vi "data_waypoint_ref.vi"() -> ()   [LabVIEW 2018] (continued)
"Y"=530253.3628541183}, {"X"=175364.75731318252, "Y"=530253.4135907482}, {"X"=175364.79603092565, "Y"=530253.4635879273}, {"X"=175364.8341888009, "Y"=530253.5129652326}, {"X"=175364.8714835971, "Y"=530253.5616292221}, {"X"=175364.90849024183, "Y"=530253.6105027163}, {"X"=175364.94563348373, "Y"=530253.6594390685}, {"X"=175364.98314331504, "Y"=530253.7089359304}, {"X"=175365.02100005752, "Y"=530253.7595272006}, {"X"=175365.05918145005, "Y"=530253.8114759818}, {"X"=175365.09803261896, "Y"=530253.864670273}, {"X"=175365.1369677881, "Y"=530253.9178143732}, {"X"=175365.175450904, "Y"=530253.9711551395}, {"X"=175365.2146263419, "Y"=530254.0234727964}, {"X"=175365.25404981908, "Y"=530254.0748962869}, {"X"=175365.29313406267, "Y"=530254.1257247813}, {"X"=175365.3311370293, "Y"=530254.1760414864}, {"X"=175365.36840857498, "Y"=530254.2258364942}, {"X"=175365.40494955413, "Y"=530254.2744971587}, {"X"=175365.44107322232, "Y"=530254.3225197739}, {"X"=175365.4766030218, "Y"=530254.3695064213}, {"X"=175365.51182505823, "Y"=530254.4166593428}, {"X"=175365.54752247653, "Y"=530254.4640172995}, {"X"=175365.58419388309, "Y"=530254.5115499632}, {"X"=175365.62093701866, "Y"=530254.5602788435}, {"X"=175365.65774631436, "Y"=530254.6098177265}, {"X"=175365.6950449408, "Y"=530254.6597857933}, {"X"=175365.73257001908, "Y"=530254.7099496393}, {"X"=175365.76995592058, "Y"=530254.7600772697}, {"X"=175365.80677752316, "Y"=530254.8101854757}, {"X"=175365.84416599848, "Y"=530254.8596838082}, {"X"=175365.88176222175, "Y"=530254.9096443404}, {"X"=175365.91953173553, "Y"=530254.9594944854}, {"X"=175365.9574402241, "Y"=530255.0090134849}, {"X"=175365.99470143978, "Y"=530255.0589117429}, {"X"=175366.03154062154, "Y"=530255.1089755029}, {"X"=175366.0680535847, "Y"=530255.1592533174}, {"X"=175366.10490100825, "Y"=530255.2091083997}, {"X"=175366.1418778741, "Y"=530255.2596034913}, {"X"=175366.1794578632, "Y"=530255.3106683819}, {"X"=175366.2173681856, "Y"=530255.3620142048}, {"X"=175366.25529422174, "Y"=530255.4138827252}, {"X"=175366.29256422166, "Y"=530255.465561172}, {"X"=175366.3293060358, "Y"=530255.517452049}, {"X"=175366.36565792985, "Y"=530255.5689833704}, {"X"=175366.40203412157, "Y"=530255.6200418209}, {"X"=175366.4388502521, "Y"=530255.6703997643}, {"X"=175366.47596965497, "Y"=530255.7205714668}, {"X"=175366.51282475406, "Y"=530255.770928185}, {"X"=175366.5496163633, "Y"=530255.821080876}, {"X"=175366.58622919343, "Y"=530255.8712851491}, {"X"=175366.62272470424, "Y"=530255.9216551357}, {"X"=175366.65895272506, "Y"=530255.9726318942}, {"X"=175366.69602994501, "Y"=530256.0244207871}, {"X"=175366.73390271078, "Y"=530256.0771507177}, {"X"=175366.77233000507, "Y"=530256.1316958538}, {"X"=175366.81173351035, "Y"=530256.1868696233}, {"X"=175366.8519770966, "Y"=530256.2427678755}, {"X"=175366.8918884384, "Y"=530256.2989401333}, {"X"=175366.93135789846, "Y"=530256.3554544192}, {"X"=175366.9706897959, "Y"=530256.4115784413}, {"X"=175367.01058779864, "Y"=530256.4677340913}, {"X"=175367.05065983246, "Y"=530256.5246328339}, {"X"=175367.09101690596, "Y"=530256.5811689214}, {"X"=175367.1310731591, "Y"=530256.6375227704}, {"X"=175367.17083612958, "Y"=530256.6932448632}, {"X"=175367.21025581684, "Y"=530256.7481999461}, {"X"=175367.2492354851, "Y"=530256.8023261506}, {"X"=175367.287581066, "Y"=530256.8564975066}, {"X"=175367.32615449073, "Y"=530256.910735893}, {"X"=175367.3651370734, "Y"=530256.9652505389}, {"X"=175367.40405244404, "Y"=530257.0192004658}, {"X"=175367.44224889282, "Y"=530257.0729627243}, {"X"=175367.48063509667, "Y"=530257.1270928971}, {"X"=175367.5193307458, "Y"=530257.1810268238}, {"X"=175367.55835376275, "Y"=530257.2354370258}, {"X"=175367.59777806984, "Y"=530257.2904586872}, {"X"=175367.63832748993, "Y"=530257.3464415018}, {"X"=175367.67939942481, "Y"=530257.4029932447}, {"X"=175367.7207491782, "Y"=530257.4600391674}, {"X"=175367.7617005033, "Y"=530257.5171439771}, {"X"=175367.80307118673, "Y"=530257.5743796235}, {"X"=175367.84486851882, "Y"=530257.6312133558}, {"X"=175367.88690845872, "Y"=530257.6877145241}, {"X"=175367.92825091735, "Y"=530257.7446905482}, {"X"=175367.9699223432, "Y"=530257.8011817061}, {"X"=175368.01151293772, "Y"=530257.8572957474}, {"X"=175368.05314487906, "Y"=530257.9130123383}, {"X"=175368.09419173302, "Y"=530257.9685697247}, {"X"=175368.13502857919, "Y"=530258.0240999819}, {"X"=175368.17578947498, "Y"=530258.0794073816}, {"X"=175368.21706993572, "Y"=530258.1336810826}, {"X"=175368.2580036735, "Y"=530258.1878248417}, {"X"=175368.29871781138, "Y"=530258.2416928933}, {"X"=175368.33960146687, "Y"=530258.29567476}, {"X"=175368.38056272513, "Y"=530258.349538754}, {"X"=175368.42160467047, "Y"=530258.403431366}, {"X"=175368.46324653408, "Y"=530258.4574065608}, {"X"=175368.50493600065, "Y"=530258.5113039257}, {"X"=175368.546039586, "Y"=530258.5653739354}, {"X"=175368.58627301786, "Y"=530258.619636295}, {"X"=175368.62661766922, "Y"=530258.6737673621}, {"X"=175368.66737663423, "Y"=530258.7275187485}, {"X"=175368.707789486, "Y"=530258.7819492777}, {"X"=175368.74817281184, "Y"=530258.8368815499}, {"X"=175368.78905969212, "Y"=530258.8922607239}, {"X"=175368.83060171016, "Y"=530258.9472239888}, {"X"=175368.87236381875, "Y"=530259.0017271258}, {"X"=175368.91362172773, "Y"=530259.0555647215}, {"X"=175368.9541187612, "Y"=530259.1088041244}, {"X"=175368.99351905257, "Y"=530259.161693824}, {"X"=175369.03251394143, "Y"=530259.2140797316}, {"X"=175369.07165795774, "Y"=530259.2668725194}, {"X"=175369.1116919916, "Y"=530259.3202020752}, {"X"=175369.1522712206, "Y"=530259.3739828493}, {"X"=175369.19244677763, "Y"=530259.4275450595}, {"X"=175369.2315454748, "Y"=530259.4811925745}, {"X"=175369.27035327113, "Y"=530259.5341139864}, {"X"=175369.30912567972, "Y"=530259.5858479531}, {"X"=175369.34761534786, "Y"=530259.637222049}, {"X"=175369.38570391198, "Y"=530259.6883464997}, {"X"=175369.4236531108, "Y"=530259.7393714729}, {"X"=175369.4617789277, "Y"=530259.7896123657}, {"X"=175369.49993611278, "Y"=530259.8390751553}, {"X"=175369.53771359075, "Y"=530259.8880362958}, {"X"=175369.57511864332, "Y"=530259.9371627924}, {"X"=175369.61242632216, "Y"=530259.9872129811}, {"X"=175369.65026476423, "Y"=530260.0379253004}, {"X"=175369.68844804208, "Y"=530260.0899329198}, {"X"=175369.72774864096, "Y"=530260.1420593341}, {"X"=175369.76747697193, "Y"=530260.1944530737}, {"X"=175369.80690045215, "Y"=530260.2470996501}, {"X"=175369.84600582987, "Y"=530260.2994086567}, {"X"=175369.8855787249, "Y"=530260.3516585723}, {"X"=175369.92548969664, "Y"=530260.4038098247}, {"X"=175369.96521553188, "Y"=530260.4568606102}, {"X"=175370.0048233524, "Y"=530260.5098418208}, {"X"=175370.04435833584, "Y"=530260.5630540976}, {"X"=175370.08360233658, "Y"=530260.6155147478}, {"X"=175370.12268043496, "Y"=530260.6666828998}, {"X"=175370.161077391, "Y"=530260.7169574014}, {"X"=175370.1988345409, "Y"=530260.7665367983}, {"X"=175370.23621340372, "Y"=530260.8160973303}, {"X"=175370.2741603868, "Y"=530260.8651700723}, {"X"=175370.31198308783, "Y"=530260.9147526048}, {"X"=175370.3494809023, "Y"=530260.9653027819}, {"X"=175370.38678381703, "Y"=530261.0161443175}, {"X"=175370.42433720775, "Y"=530261.0678208391}, {"X"=175370.4626341092, "Y"=530261.1193120438}, {"X"=175370.50168795633, "Y"=530261.1715712609}, {"X"=175370.54076009642, "Y"=530261.2252288469}, {"X"=175370.58048902013, "Y"=530261.279631433}, {"X"=175370.62107124308, "Y"=530261.333832843}, {"X"=175370.66210860672, "Y"=530261.3879840766}, {"X"=175370.70264565348, "Y"=530261.4421856187}, {"X"=175370.74249817466, "Y"=530261.4961483381}, {"X"=175370.78169428193, "Y"=530261.5497933521}, {"X"=175370.82119589235, "Y"=530261.6028059552}, {"X"=175370.8604972166, "Y"=530261.6560855159}, {"X"=175370.89999125095, "Y"=530261.7092335463}, {"X"=175370.93876096676, "Y"=530261.7621650669}, {"X"=175370.97771263926, "Y"=530261.8146221417}, {"X"=175371.01739352918, "Y"=530261.8662513338}, {"X"=175371.057154059, "Y"=530261.9175528833}, {"X"=175371.09605709632, "Y"=530261.9691366423}, {"X"=175371.13461257404, "Y"=530262.0218090902}, {"X"=175371.17493162048, "Y"=530262.074476341}, {"X"=175371.2161687712, "Y"=530262.1281930344}, {"X"=175371.2574986481, "Y"=530262.1824155508}, {"X"=175371.29896848748, "Y"=530262.2372436394}, {"X"=175371.34017383057, "Y"=530262.2927928045}, {"X"=175371.38163837852, "Y"=530262.3479305593}, {"X"=175371.4233859332, "Y"=530262.4026168778}, {"X"=175371.4653806578, "Y"=530262.457616558}, {"X"=175371.50709616198, "Y"=530262.5134505647}, {"X"=175371.5492311775, "Y"=530262.5688660291}, {"X"=175371.59135206408, "Y"=530262.6242970738}, {"X"=175371.63361993022, "Y"=530262.6797065984}, {"X"=175371.67533013487, "Y"=530262.7352465111}, {"X"=175371.7166030467, "Y"=530262.7908820468}, {"X"=175371.7576439664, "Y"=530262.846846788}, {"X"=175371.79961031346, "Y"=530262.9018365643}, {"X"=175371.8417403082, "Y"=530262.9558502925}, {"X"=175371.88340146284, "Y"=530263.0091728515}, {"X"=175371.92439824372, "Y"=530263.0615795128}, {"X"=175371.96503316762, "Y"=530263.1135310883}, {"X"=175372.0052249805, "Y"=530263.1648058448}, {"X"=175372.04496494954, "Y"=530263.216047527}, {"X"=175372.08486382675, "Y"=530263.267409716}, {"X"=175372.12527531054, "Y"=530263.3195872516}, {"X"=175372.16591554228, "Y"=530263.3718373646}, {"X"=175372.20672269005, "Y"=530263.4245209418}, {"X"=175372.24767576595, "Y"=530263.4771275077}, {"X"=175372.28965336786, "Y"=530263.5290240761}, {"X"=175372.33110264182, "Y"=530263.5816868937}, {"X"=175372.3726853523, "Y"=530263.6348432075}, {"X"=175372.4151099726, "Y"=530263.6881424303}, {"X"=175372.45798269208, "Y"=530263.7411051576}, {"X"=175372.50007205043, "Y"=530263.7942555395}, {"X"=175372.5416247459, "Y"=530263.8474474571}, {"X"=175372.5829580622, "Y"=530263.9010406794}, {"X"=175372.62484024334, "Y"=530263.9542238587}, {"X"=175372.66669413337, "Y"=530264.0071252142}, {"X"=175372.70904192966, "Y"=530264.0599052535}, {"X"=175372.75097860975, "Y"=530264.112345775}, {"X"=175372.7924628684, "Y"=530264.1645578903}, {"X"=175372.8333104372, "Y"=530264.2162313784}, {"X"=175372.8738449646, "Y"=530264.2680833666}, {"X"=175372.91441410081, "Y"=530264.319957451}, {"X"=175372.9557862025, "Y"=530264.3719834397}, {"X"=175372.99767016945, "Y"=530264.4239701862}, {"X"=175373.03924414562, "Y"=530264.4765704875}, {"X"=175373.0804756962, "Y"=530264.529296102}, {"X"=175373.12245933426, "Y"=530264.5811404951}, {"X"=175373.1641074646, "Y"=530264.6327539145}, {"X"=175373.2048067197, "Y"=530264.6842968779}, {"X"=175373.245243158, "Y"=530264.7356275225}, {"X"=175373.28613031158, "Y"=530264.7872098872}, {"X"=175373.3268719919, "Y"=530264.8396239675}, {"X"=175373.36816244232, "Y"=530264.8921995794}, {"X"=175373.40948345076, "Y"=530264.9443233894}, {"X"=175373.45060314657, "Y"=530264.9963656624}, {"X"=175373.49133239881, "Y"=530265.0475689222}, {"X"=175373.53206551704, "Y"=530265.0985812743}, {"X"=175373.5723972954, "Y"=530265.1501674973}, {"X"=175373.6127379377, "Y"=530265.2029590018}, {"X"=175373.65307959612, "Y"=530265.2560956681}, {"X"=175373.6935509451, "Y"=530265.3090554855}, {"X"=175373.73412274377, "Y"=530265.3609340055}, {"X"=175373.7750503279, "Y"=530265.4118103823}, {"X"=175373.8156763603, "Y"=530265.4625544671}, {"X"=175373.85636513907, "Y"=530265.512649098}, {"X"=175373.8966237603, "Y"=530265.5631567544}, {"X"=175373.9368359794, "Y"=530265.6141495564}, {"X"=175373.97664394762, "Y"=530265.6659315486}, {"X"=175374.01652882574, "Y"=530265.7176611514}, {"X"=175374.0558253849, "Y"=530265.7696377665}, {"X"=175374.09546728528, "Y"=530265.8215756294}, {"X"=175374.1352996199, "Y"=530265.8735107117}, {"X"=175374.1753605969, "Y"=530265.9263862808}, {"X"=175374.21554098636, "Y"=530265.9792048966}, {"X"=175374.25634345112, "Y"=530266.0321115775}, {"X"=175374.29684755186, "Y"=530266.0847660915}, {"X"=175374.3370072678, "Y"=530266.1368822271}, {"X"=175374.37684985562, "Y"=530266.1883899836}, {"X"=175374.41664284474, "Y"=530266.2401997693}, {"X"=175374.45623583646, "Y"=530266.2926760602}, {"X"=175374.4957903801, "Y"=530266.3453322599}, {"X"=175374.53494277128, "Y"=530266.3985856391}, {"X"=175374.5738609444, "Y"=530266.4514124128}, {"X"=175374.61273645412, "Y"=530266.5035878264}, {"X"=175374.6511642197, "Y"=530266.5553183937}, {"X"=175374.68891586334, "Y"=530266.6066558418}, {"X"=175374.72739777548, "Y"=530266.6569223469}, {"X"=175374.7656299184, "Y"=530266.7065947026}, {"X"=175374.80313963493, "Y"=530266.7566920433}, {"X"=175374.8399778119, "Y"=530266.8064484142}, {"X"=175374.8766657008, "Y"=530266.8563062254}, {"X"=175374.91344849125, "Y"=530266.9059040511}, {"X"=175374.95023190015, "Y"=530266.9560135192}, {"X"=175374.98740198716, "Y"=530267.0068876502}, {"X"=175375.02601149524, "Y"=530267.0580716352}, {"X"=175375.06553802377, "Y"=530267.1114426706}, {"X"=175375.10591067414, "Y"=530267.1669876481}, {"X"=175375.146517546, "Y"=530267.2238637658}, {"X"=175375.1877406851, "Y"=530267.2809611515}, {"X"=175375.22830013547, "Y"=530267.3382780246}, {"X"=175375.26785239112, "Y"=530267.3949719046}, {"X"=175375.30721058228, "Y"=530267.4504355218}, {"X"=175375.34715167427, "Y"=530267.5053180757}, {"X"=175375.38706773933, "Y"=530267.5595225785}, {"X"=175375.4267418654, "Y"=530267.613685621}, {"X"=175375.46535510637, "Y"=530267.6676442431}, {"X"=175375.50396058234, "Y"=530267.7216716999}, {"X"=175375.54284507962, "Y"=530267.7750990131}, {"X"=175375.58147326022, "Y"=530267.8287157561}, {"X"=175375.61925587003, "Y"=530267.8830519565}, {"X"=175375.6576886122, "Y"=530267.9376803568}, {"X"=175375.69664500767, "Y"=530267.9926623688}, {"X"=175375.73603756493, "Y"=530268.0480681743}, {"X"=175375.77532893803, "Y"=530268.1040047903}, {"X"=175375.81435740308, "Y"=530268.1602995562}, {"X"=175375.85262212646, "Y"=530268.2171293042}, {"X"=175375.89158039243, "Y"=530268.2739503484}, {"X"=175375.93173150255, "Y"=530268.330970986}, {"X"=175375.97191079802, "Y"=530268.3882379278}, {"X"=175376.01228297348, "Y"=530268.4463333681}, {"X"=175376.05265943654, "Y"=530268.5043810724}, {"X"=175376.09293965067, "Y"=530268.562530056}, {"X"=175376.13402299516, "Y"=530268.6205878863}, {"X"=175376.17550761972, "Y"=530268.6789541855}, {"X"=175376.2171191087, "Y"=530268.7382901298}, {"X"=175376.25857909265, "Y"=530268.798215855}, {"X"=175376.30063365336, "Y"=530268.8576137554}, {"X"=175376.34250984906, "Y"=530268.9169023044}, {"X"=175376.38375533113, "Y"=530268.9761782852}, {"X"=175376.4239993277, "Y"=530269.0352652095}, {"X"=175376.46462206956, "Y"=530269.0942278227}, {"X"=175376.5061171255, "Y"=530269.1522278391}, {"X"=175376.5475091983, "Y"=530269.20984859}, {"X"=175376.58769639168, "Y"=530269.2676948581}, {"X"=175376.62757688668, "Y"=530269.3254665607}, {"X"=175376.667320457, "Y"=530269.3824628744}, {"X"=175376.70731428557, "Y"=530269.4393174993}, {"X"=175376.74719239495, "Y"=530269.495980459}, {"X"=175376.7866007532, "Y"=530269.5537480027}, {"X"=175376.82704140185, "Y"=530269.6116368113}, {"X"=175376.86867427992, "Y"=530269.6692157873}, {"X"=175376.91032201465, "Y"=530269.7264251373}, {"X"=175376.9512818232, "Y"=530269.7837452792}, {"X"=175376.99105095697, "Y"=530269.8410012267}, {"X"=175377.02996204546, "Y"=530269.8986514817}, {"X"=175377.06897030905, "Y"=530269.9562137703}, {"X"=175377.1089557823, "Y"=530270.0135423321}, {"X"=175377.14928842592, "Y"=530270.0708510028}, {"X"=175377.18985192844, "Y"=530270.1274475757}, {"X"=175377.2301206264, "Y"=530270.1834967455}, {"X"=175377.2706423454, "Y"=530270.2388393001}, {"X"=175377.31043959537, "Y"=530270.2942139549}, {"X"=175377.34961013673, "Y"=530270.3497336272}, {"X"=175377.38805029093, "Y"=530270.4062842885}, {"X"=175377.42698760645, "Y"=530270.4629167287}, {"X"=175377.4664671266, "Y"=530270.5195853052}, {"X"=175377.50645504915, "Y"=530270.5753411908}, {"X"=175377.5459466516, "Y"=530270.6313005314}, {"X"=175377.58575752817, "Y"=530270.6876951077}, {"X"=175377.62575899236, "Y"=530270.7447406121}, {"X"=175377.66585884744, "Y"=530270.8024117845}, {"X"=175377.70568216513, "Y"=530270.8603246126}, {"X"=175377.74558738028, "Y"=530270.9180740495}, {"X"=175377.7855966506, "Y"=530270.974763265}, {"X"=175377.82569728378, "Y"=530271.0302924092}, {"X"=175377.86556871625, "Y"=530271.084692392}, {"X"=175377.90532123862, "Y"=530271.1393202449}, {"X"=175377.94501325546, "Y"=530271.1944565923}, {"X"=175377.98486513883, "Y"=530271.2503405145}, {"X"=175378.02435570536, "Y"=530271.3062510273}, {"X"=175378.06409336728, "Y"=530271.3621497148}, {"X"=175378.103309077, "Y"=530271.4176703686}, {"X"=175378.14220560313, "Y"=530271.473087634}, {"X"=175378.1814429543, "Y"=530271.5284373041}, {"X"=175378.22134028416, "Y"=530271.5838127786}, {"X"=175378.26121354155, "Y"=530271.6397365938}, {"X"=175378.30082891998, "Y"=530271.695920876}, {"X"=175378.34050395305, "Y"=530271.7519096485}, {"X"=175378.38047696327, "Y"=530271.8074180826}, {"X"=175378.42039218737, "Y"=530271.8628545483}, {"X"=175378.46029272696, "Y"=530271.9181179173}, {"X"=175378.50024812756, "Y"=530271.973962691}, {"X"=175378.54103024217, "Y"=530272.0296030378}, {"X"=175378.58160302788, "Y"=530272.0854482147}, {"X"=175378.6219478474, "Y"=530272.1405826434}, {"X"=175378.66133265817, "Y"=530272.1948741865}, {"X"=175378.70041345863, "Y"=530272.2478991648}, {"X"=175378.73875308977, "Y"=530272.3003991435}, {"X"=175378.7769726777, "Y"=530272.3530437571}, {"X"=175378.81478900305, "Y"=530272.4059093122}, {"X"=175378.85344642977, "Y"=530272.4595459604}, {"X"=175378.8927827093, "Y"=530272.5129997034}, {"X"=175378.9328368426, "Y"=530272.5662793056}, {"X"=175378.97299077566, "Y"=530272.619159064}, {"X"=175379.01313879451, "Y"=530272.6724361693}, {"X"=175379.05281503018, "Y"=530272.7267301857}, {"X"=175379.09275090517, "Y"=530272.7819634884}, {"X"=175379.13273609988, "Y"=530272.8380035125}, {"X"=175379.17377965036, "Y"=530272.8933911546}, {"X"=175379.21499514012, "Y"=530272.9488104766}, {"X"=175379.25621501883, "Y"=530273.0033163701}, {"X"=175379.2960237182, "Y"=530273.0580761392}, {"X"=175379.33575262167, "Y"=530273.1128117243}, {"X"=175379.3756350914, "Y"=530273.1676578454}, {"X"=175379.41577269154, "Y"=530273.222211321}, {"X"=175379.45561149748, "Y"=530273.2769687815}, {"X"=175379.49584439732, "Y"=530273.3307983498}, {"X"=175379.53572220702, "Y"=530273.3837610537}, {"X"=175379.57504594701, "Y"=530273.4362681268}, {"X"=175379.61395791481, "Y"=530273.4879118324}, {"X"=175379.653285014, "Y"=530273.5397552007}, {"X"=175379.69188306064, "Y"=530273.5924819438}, {"X"=175379.73056062285, "Y"=530273.6460419565}, {"X"=175379.76959291293, "Y"=530273.6994422176}, {"X"=175379.8094673134, "Y"=530273.7524515456}, {"X"=175379.8491786922, "Y"=530273.8051483744}, {"X"=175379.88896082636, "Y"=530273.8581091418}, {"X"=175379.9291784505, "Y"=530273.9121673888}, {"X"=175379.97054167185, "Y"=530273.9666229206}, {"X"=175380.01182172928, "Y"=530274.0226169619}, {"X"=175380.05318232844, "Y"=530274.079491995}, {"X"=175380.09513207295, "Y"=530274.1364019196}, {"X"=175380.13819652947, "Y"=530274.1925460887}, {"X"=175380.18149366078, "Y"=530274.2491956674}, {"X"=175380.2250484434, "Y"=530274.3055070925}, {"X"=175380.26838144008, "Y"=530274.3623041774}, {"X"=175380.31188147655, "Y"=530274.4186745853}, {"X"=175380.3549409229, "Y"=530274.4749230964}, {"X"=175380.3972649774, "Y"=530274.5308053015}, {"X"=175380.43836973322, "Y"=530274.5862271729}, {"X"=175380.47931384272, "Y"=530274.6406384385}, {"X"=175380.5204471117, "Y"=530274.694614081}, {"X"=175380.56209510507, "Y"=530274.748920056}, {"X"=175380.60371871642, "Y"=530274.8033692753}, {"X"=175380.6451534636, "Y"=530274.8583540027}, {"X"=175380.68621689494, "Y"=530274.91297912}, {"X"=175380.72710987853, "Y"=530274.9677778766}, {"X"=175380.76810750342, "Y"=530275.0226162815}, {"X"=175380.80994694738, "Y"=530275.0778672938}, {"X"=175380.85239067252, "Y"=530275.1334805603}, {"X"=175380.89503053552, "Y"=530275.1901265308}, {"X"=175380.9377349384, "Y"=530275.246731244}, {"X"=175380.9805978658, "Y"=530275.3030247326}, {"X"=175381.0230490275, "Y"=530275.3587578452}, {"X"=175381.06513342983, "Y"=530275.4135730725}, {"X"=175381.10631238978, "Y"=530275.4686295863}, {"X"=175381.14743795973, "Y"=530275.5233022464}, {"X"=175381.18891169218, "Y"=530275.5779927488}, {"X"=175381.23041948982, "Y"=530275.6325200024}, {"X"=175381.27197850702, "Y"=530275.6875975949}, {"X"=175381.3141971989, "Y"=530275.7425955562}, {"X"=175381.35612077633, "Y"=530275.7987464201}, {"X"=175381.39866254883, "Y"=530275.8545702754}, {"X"=175381.44144096706, "Y"=530275.9110449206}, {"X"=175381.48396489912, "Y"=530275.9674281975}, {"X"=175381.52566846483, "Y"=530276.0237661658}, {"X"=175381.56639495818, "Y"=530276.0791813901}, {"X"=175381.60614632058, "Y"=530276.1337315745}, {"X"=175381.64565829624, "Y"=530276.1873035681}, {"X"=175381.68537671026, "Y"=530276.2408927118}, {"X"=175381.72567720927, "Y"=530276.2954279619}, {"X"=175381.76592636586, "Y"=530276.3505771153}, {"X"=175381.8065536897, "Y"=530276.4066074943}, {"X"=175381.84723761232, "Y"=530276.4623069686}, {"X"=175381.8881185681, "Y"=530276.5175375018}, {"X"=175381.92892906343, "Y"=530276.5717005575}, {"X"=175381.96981449414, "Y"=530276.6260454104}, {"X"=175382.0109063195, "Y"=530276.6806926475}, {"X"=175382.05228986236, "Y"=530276.7360426767}, {"X"=175382.09401500106, "Y"=530276.7918878068}, {"X"=175382.13590830663, "Y"=530276.848290703}, {"X"=175382.17683812688, "Y"=530276.9053778878}, {"X"=175382.21736197197, "Y"=530276.9623663815}, {"X"=175382.25794670594, "Y"=530277.0195777777}, {"X"=175382.299110183, "Y"=530277.076300242}, {"X"=175382.3405598369, "Y"=530277.1330462806}, {"X"=175382.3816216344, "Y"=530277.1898323065}, {"X"=175382.42177914153, "Y"=530277.246647631}, {"X"=175382.4623105062, "Y"=530277.3016794228}, {"X"=175382.50294386526, "Y"=530277.3558518823}, {"X"=175382.54306338512, "Y"=530277.4093932352}, {"X"=175382.58212770906, "Y"=530277.4634571102}, {"X"=175382.62030600384, "Y"=530277.5183382287}, {"X"=175382.65887284116, "Y"=530277.5734135413}, {"X"=175382.69841257622, "Y"=530277.6285958623}, {"X"=175382.73787164403, "Y"=530277.6837573361}, {"X"=175382.77683788392, "Y"=530277.7388048348}, {"X"=175382.81560297194, "Y"=530277.7935244082}, {"X"=175382.85500985917, "Y"=530277.8484130106}, {"X"=175382.89468581765, "Y"=530277.9029312362}, {"X"=175382.93342362894, "Y"=530277.9580138144}, {"X"=175382.97016422707, "Y"=530278.0137726283}, {"X"=175383.00719641265, "Y"=530278.0689867527}, {"X"=175383.04524049233, "Y"=530278.1234110076}, {"X"=175383.08446525745, "Y"=530278.177516587}, {"X"=175383.12400785997, "Y"=530278.2324713808}, {"X"=175383.16341338272, "Y"=530278.2884021463}, {"X"=175383.20321088587, "Y"=530278.3450931216}, {"X"=175383.24388467334, "Y"=530278.4018691962}, {"X"=175383.28416762798, "Y"=530278.46038113}, {"X"=175383.32348511857, "Y"=530278.5201078751}, {"X"=175383.36322165257, "Y"=530278.5798589126}, {"X"=175383.40385465274, "Y"=530278.6390279633}, {"X"=175383.44465535972, "Y"=530278.6989001713}, {"X"=175383.4862341692, "Y"=530278.75830284}, {"X"=175383.52822093136, "Y"=530278.8175722327}, {"X"=175383.56995807827, "Y"=530278.8769011825}, {"X"=175383.61148408483, "Y"=530278.9361197695}, {"X"=175383.65323525056, "Y"=530278.9944953114}, {"X"=175383.69421530858, "Y"=530279.0530074155}, {"X"=175383.7350554744, "Y"=530279.111541019}, {"X"=175383.77542995836, "Y"=530279.1704555652}, {"X"=175383.8157298488, "Y"=530279.2293070713}, {"X"=175383.8559401721, "Y"=530279.2881233235}, {"X"=175383.89695070562, "Y"=530279.3461569902}, {"X"=175383.93826252603, "Y"=530279.4039311717}, {"X"=175383.97949878522, "Y"=530279.4619153388}, {"X"=175384.02036026714, "Y"=530279.5201691986}, {"X"=175384.06054778706, "Y"=530279.5790632094}, {"X"=175384.10039149693, "Y"=530279.6382146104}, {"X"=175384.14101006766, "Y"=530279.6973004678}, {"X"=175384.1822571442, "Y"=530279.7559505224}, {"X"=175384.22384488, "Y"=530279.8141767163}, {"X"=175384.26575571846, "Y"=530279.8720312649}, {"X"=175384.30757643149, "Y"=530279.9302634323}, {"X"=175384.34938070193, "Y"=530279.988026178}, {"X"=175384.39056756336, "Y"=530280.0457807535}, {"X"=175384.4300316461, "Y"=530280.1038567104}, {"X"=175384.46858665868, "Y"=530280.1612416819}, {"X"=175384.5074643027, "Y"=530280.2174947566}, {"X"=175384.54749630456, "Y"=530280.2726090478}, {"X"=175384.586673461, "Y"=530280.3276992185}, {"X"=175384.62548891825, "Y"=530280.3817849228}, {"X"=175384.66357065516, "Y"=530280.4351669155}, {"X"=175384.70142916602, "Y"=530280.4873442599}, {"X"=175384.7383800607, "Y"=530280.538421075}, {"X"=175384.77384348479, "Y"=530280.5882103939}, {"X"=175384.80759560052, "Y"=530280.6358982379}, {"X"=175384.8404099675, "Y"=530280.6812770056}, {"X"=175384.87250879448, "Y"=530280.7243071992}, {"X"=175384.90436964578, "Y"=530280.7647299246}, {"X"=175384.93436790677, "Y"=530280.80311488}, {"X"=175384.9616378935, "Y"=530280.8381638632}, {"X"=175384.9850736076, "Y"=530280.8648757731}, {"X"=175385.00324402758, "Y"=530280.8833868961}, {"X"=175385.0150459357, "Y"=530280.8944529634}, {"X"=175385.02297698648, "Y"=530280.9010033109}, {"X"=175385.02939790592, "Y"=530280.9042851299}, {"X"=175385.03577591613, "Y"=530280.9056281495}, {"X"=175385.04157625238, "Y"=530280.9066199363}, {"X"=175385.04734175224, "Y"=530280.9069115034}, {"X"=175385.0522705122, "Y"=530280.9070113084}, {"X"=175385.05647557072, "Y"=530280.9068024849}, {"X"=175385.06001046783, "Y"=530280.9061183934}, {"X"=175385.06346903727, "Y"=530280.9044811573}, {"X"=175385.06641534183, "Y"=530280.9021439983}, {"X"=175385.06904727407, "Y"=530280.8992328586}, {"X"=175385.0711258982, "Y"=530280.896123573}, {"X"=175385.0733705323, "Y"=530280.8925376674}, {"X"=175385.0755269345, "Y"=530280.8887688976}, {"X"=175385.07764847262, "Y"=530280.8848914615}, {"X"=175385.07942518912, "Y"=530280.8812292453}, {"X"=175385.08167830165, "Y"=530280.8775145715}, {"X"=175385.08414133126, "Y"=530280.8740967229}, {"X"=175385.08691378706, "Y"=530280.871078623}]
  in  "length":i32=760
  in  "정지":bool
  out "part length":i32=3762
  out "way point":cluster{"X":dbl, "Y":dbl}[](graph)=[{"X"=175269.23338394496, "Y"=530125.5650971091}, {"X"=175269.23350506835, "Y"=530125.5650190613}, {"X"=175269.2336243907, "Y"=530125.5649310285}, {"X"=175269.23374547902, "Y"=530125.5648418807}, {"X"=175269.2338656248, "Y"=530125.5647327604}, {"X"=175269.23387002628, "Y"=530125.564722758}, {"X"=175269.23380981, "Y"=530125.564729596}, {"X"=175269.23373898986, "Y"=530125.5647442333}, {"X"=175269.23368053322, "Y"=530125.5647455158}, {"X"=175269.23362026666, "Y"=530125.5647345963}, {"X"=175269.23355642756, "Y"=530125.5647136965}, {"X"=175269.23348461336, "Y"=530125.5646917124}, {"X"=175269.2334322464, "Y"=530125.5646563518}, {"X"=175269.2333984662, "Y"=530125.5646153864}, {"X"=175269.2333726424, "Y"=530125.5645699587}, {"X"=175269.23333709498, "Y"=530125.5645312194}, {"X"=175269.23331302856, "Y"=530125.5644802372}, {"X"=175269.23329159417, "Y"=530125.5644214775}, {"X"=175269.23327721853, "Y"=530125.5643527095}, {"X"=175269.23325133463, "Y"=530125.5642861942}, {"X"=175269.23324577717, "Y"=530125.564204081}, {"X"=175269.23325435573, "Y"=530125.5641097176}, {"X"=175269.23326999962, "Y"=530125.5640075641}, {"X"=175269.23327324167, "Y"=530125.5639065579}, {"X"=175269.2332826196, "Y"=530125.563782226}, {"X"=175269.23324711813, "Y"=530125.563759023}, {"X"=175269.2332064203, "Y"=530125.5637757913}, {"X"=175269.23316041677, "Y"=530125.5637947962}, {"X"=175269.2331205653, "Y"=530125.5637982432}, {"X"=175269.23308069742, "Y"=530125.5637961407}, {"X"=175269.23303194798, "Y"=530125.5637851872}, {"X"=175269.23297789812, "Y"=530125.5637797968}, {"X"=175269.2329237925, "Y"=530125.5637555401}, {"X"=175269.2328661067, "Y"=530125.5637179757}, {"X"=175269.23281019018, "Y"=530125.5636804058}, {"X"=175269.2327534404, "Y"=530125.5636605966}, {"X"=175269.23269399066, "Y"=530125.5636263662}, {"X"=175269.2326309815, "Y"=530125.5635865974}, {"X"=175269.2325608896, "Y"=530125.5635479597}, {"X"=175269.23248814695, "Y"=530125.5635115493}, {"X"=175269.23242423232, "Y"=530125.563465125}, {"X"=175269.2323682567, "Y"=530125.5634075777}, {"X"=175269.2323122811, "Y"=530125.5633500303}, {"X"=175269.2322554394, "Y"=530125.5632991446}, {"X"=175269.23220741484, "Y"=530125.5632338051}, {"X"=175269.23217642424, "Y"=530125.5632383368}, {"X"=175269.23216853777, "Y"=530125.5632672162}, {"X"=175269.23216774064, "Y"=530125.5632971842}, {"X"=175269.23216602165, "Y"=530125.5633149485}, {"X"=175269.2321758175, "Y"=530125.5633326776}, {"X"=175269.23219005423, "Y"=530125.5633537214}, {"X"=175269.23221757179, "Y"=530125.5633736176}, {"X"=175269.2322476908, "Y"=530125.5633746382}, {"X"=175269.2322830872, "Y"=530125.5633623255}, {"X"=175269.23231138548, "Y"=530125.5633467035}, {"X"=175269.2323450038, "Y"=530125.5633321772}, {"X"=175269.23238299944, "Y"=530125.5633009868}, {"X"=175269.23244134674, "Y"=530125.5632619705}, {"X"=175269.2325014656, "Y"=530125.5632229473}, {"X"=175269.23257220365, "Y"=530125.5631805635}, {"X"=175269.2326526489, "Y"=530125.5631259418}, {"X"=175269.2327392715, "Y"=530125.563063533}, {"X"=175269.23282324238, "Y"=530125.5630022436}, {"X"=175269.23290721097, "Y"=530125.562940952}, {"X"=175269.23300000106, "Y"=530125.5628674282}, {"X"=175269.23301239734, "Y"=530125.5628651711}, {"X"=175269.23298057573, "Y"=530125.5628874622}, {"X"=175269.2329434636, "Y"=530125.5629186487}, {"X"=175269.23292137324, "Y"=530125.5629375814}, {"X"=175269.2329063679, "Y"=530125.5629553832}, {"X"=175269.23289402967, "Y"=530125.5629765069}, {"X"=175269.23288527058, "Y"=530125.5630098284}, {"X"=175269.23302134182, "Y"=530125.563194773}, {"X"=175269.23375932508, "Y"=530125.5641326404}, {"X"=175269.23549232722, "Y"=530125.5663594418}, {"X"=175269.23821299706, "Y"=530125.5697886285}, {"X"=175269.2418305139, "Y"=530125.5742573208}, {"X"=175269.24613400537, "Y"=530125.5794509418}, {"X"=175269.2510283491, "Y"=530125.5855528992}, {"X"=175269.25636849433, "Y"=530125.5926357633}, {"X"=175269.2621807428, "Y"=530125.6003098963}, {"X"=175269.26839897686, "Y"=530125.6080827157}, {"X"=175269.2745872489, "Y"=530125.6156081256}, {"X"=175269.2805345916, "Y"=530125.6231353587}, {"X"=175269.2865490844, "Y"=530125.6306057886}, {"X"=175269.292527625, "Y"=530125.6378998575}, {"X"=175269.29843938188, "Y"=530125.6453761411}, {"X"=175269.30474220664, "Y"=530125.6535959848}, {"X"=175269.31187188625, "Y"=530125.6625547678}, {"X"=175269.31984950454, "Y"=530125.6718917236}, {"X"=175269.3283769464, "Y"=530125.68174092}, {"X"=175269.3370058783, "Y"=530125.6920615049}, {"X"=175269.34517321878, "Y"=530125.7029505935}, {"X"=175269.35338396515, "Y"=530125.7141403252}, {"X"=175269.3621428922, "Y"=530125.7249865998}, {"X"=175269.3718555859, "Y"=530125.7360542445}, {"X"=175269.38209727049, "Y"=530125.7483777951}, {"X"=175269.3927331287, "Y"=530125.7621962687}, {"X"=175269.40442856954, "Y"=530125.7772724102}, {"X"=175269.41734235984, "Y"=530125.792776682}, {"X"=175269.43073834633, "Y"=530125.8086901787}, {"X"=175269.4441001964, "Y"=530125.8253407187}, {"X"=175269.45822637147, "Y"=530125.8422520371}, {"X"=175269.47279883805, "Y"=530125.8597125255}, {"X"=175269.48706333336, "Y"=530125.8784669102}, {"X"=175269.50215967646, "Y"=530125.8978492357}, {"X"=175269.5182151948, "Y"=530125.9168857752}, {"X"=175269.53417372837, "Y"=530125.9366739778}, {"X"=175269.55044428425, "Y"=530125.9568375006}, {"X"=175269.5668258805, "Y"=530125.9765079169}, {"X"=175269.58289700188, "Y"=530125.9966265246}, {"X"=175269.59910273366, "Y"=530126.0164361936}, {"X"=175269.61485481312, "Y"=530126.03620281}, {"X"=175269.63065302302, "Y"=530126.0565908109}, {"X"=175269.64748283898, "Y"=530126.0765640037}, {"X"=175269.6643076504, "Y"=530126.0969423088}, {"X"=175269.68164738783, "Y"=530126.1186120764}, {"X"=175269.69983351757, "Y"=530126.141335929}, {"X"=175269.7193804372, "Y"=530126.1662266385}, {"X"=175269.7414211454, "Y"=530126.1933086056}, {"X"=175269.76533270563, "Y"=530126.2234038551}, {"X"=175269.79090560033, "Y"=530126.2566528512}, {"X"=175269.81794851515, "Y"=530126.2921638312}, {"X"=175269.84636353442, "Y"=530126.3285752885}, {"X"=175269.87526527036, "Y"=530126.365427031}, {"X"=175269.9045234816, "Y"=530126.4015119143}, {"X"=175269.93421858508, "Y"=530126.4367642237}, {"X"=175269.9631408176, "Y"=530126.4718612174}, {"X"=175269.99094034248, "Y"=530126.5071213518}, {"X"=175270.01842583815, "Y"=530126.5413269402}, {"X"=175270.04545693292, "Y"=530126.5746382147}, {"X"=175270.07173683835, "Y"=530126.6073390684}, {"X"=175270.09756362764, "Y"=530126.6389802392}, {"X"=175270.1229966995, "Y"=530126.6698789683}, {"X"=175270.1481672012, "Y"=530126.7003522854}, {"X"=175270.17318475395, "Y"=530126.7312233876}, {"X"=175270.19833633373, "Y"=530126.7627855352}, {"X"=175270.2241906921, "Y"=530126.7950625714}, {"X"=175270.25023147376, "Y"=530126.8286764381}, {"X"=175270.27732534253, "Y"=530126.8631473319}, {"X"=175270.30570408734, "Y"=530126.8986765608}, {"X"=175270.33564150287, "Y"=530126.9355929405}, {"X"=175270.36689411936, "Y"=530126.9745375847}, {"X"=175270.39963815565, "Y"=530127.0154911029}, {"X"=175270.43374836806, "Y"=530127.0580376677}, {"X"=175270.46832037304, "Y"=530127.1015828503}, {"X"=175270.50288421873, "Y"=530127.1450647956}, {"X"=175270.53747887694, "Y"=530127.1881826138}, {"X"=175270.57192828765, "Y"=530127.23100786}, {"X"=175270.60642698483, "Y"=530127.2728285393}, {"X"=175270.64044317373, "Y"=530127.31413456}, {"X"=175270.67375797432, "Y"=530127.3551951571}, {"X"=175270.70653323358, "Y"=530127.3956247304}, {"X"=175270.7386976343, "Y"=530127.4358718732}, {"X"=175270.77095326435, "Y"=530127.4752153223}, {"X"=175270.803546783, "Y"=530127.5131993024}, {"X"=175270.83556342172, "Y"=530127.5511050817}, {"X"=175270.86706782103, "Y"=530127.5889258045}, {"X"=175270.898346829, "Y"=530127.6263132413}, {"X"=175270.92873091088, "Y"=530127.6642060897}, {"X"=175270.95906360378, "Y"=530127.7017960993}, {"X"=175270.98970322256, "Y"=530127.739535032}, {"X"=175271.02088969247, "Y"=530127.7779793275}, {"X"=175271.05318131382, "Y"=530127.8163160286}, {"X"=175271.08623127558, "Y"=530127.8546871112}, {"X"=175271.11904272687, "Y"=530127.8938779756}, {"X"=175271.1518080221, "Y"=530127.9330379019}, {"X"=175271.1847880097, "Y"=530127.971709965}, {"X"=175271.2175635835, "Y"=530128.0101517801}, {"X"=175271.24993272143, "Y"=530128.0480431995}, {"X"=175271.28189309163, "Y"=530128.0857937655}, {"X"=175271.31334640068, "Y"=530128.1237134187}, {"X"=175271.34426640585, "Y"=530128.1616135638}, {"X"=175271.37529935152, "Y"=530128.1996654245}, {"X"=175271.40669261958, "Y"=530128.2382489524}, {"X"=175271.43880531946, "Y"=530128.2762898505}, {"X"=175271.47128172842, "Y"=530128.3136138156}, {"X"=175271.5031661289, "Y"=530128.3511359749}, {"X"=175271.5347820337, "Y"=530128.3883248628}, {"X"=175271.56640480342, "Y"=530128.4248400442}, {"X"=175271.59770678927, "Y"=530128.4610132286}, {"X"=175271.62930215636, "Y"=530128.497248809}, {"X"=175271.66133578197, "Y"=530128.5343110458}, {"X"=175271.69323693422, "Y"=530128.5730062777}, {"X"=175271.72590114985, "Y"=530128.6124328702}, {"X"=175271.75902261987, "Y"=530128.6522221451}, {"X"=175271.79217990715, "Y"=530128.692142277}, {"X"=175271.82556430704, "Y"=530128.7315811696}, {"X"=175271.858756607, "Y"=530128.7704601516}, {"X"=175271.89182269666, "Y"=530128.8082962362}, {"X"=175271.92457674904, "Y"=530128.8454540124}, {"X"=175271.95688284995, "Y"=530128.8821003588}, {"X"=175271.9887755214, "Y"=530128.9185270657}, {"X"=175272.02104236395, "Y"=530128.9550780789}, {"X"=175272.05388728023, "Y"=530128.9918094015}, {"X"=175272.08653642237, "Y"=530129.0288365249}, {"X"=175272.11878299102, "Y"=530129.0660202195}, {"X"=175272.15098487114, "Y"=530129.1030686443}, {"X"=175272.1830520333, "Y"=530129.1397922768}, {"X"=175272.2146095839, "Y"=530129.1764208594}, {"X"=175272.2457107406, "Y"=530129.2129786522}, {"X"=175272.27716318905, "Y"=530129.2500104259}, {"X"=175272.3097917369, "Y"=530129.2869632497}, {"X"=175272.34374056378, "Y"=530129.3240675495}, {"X"=175272.3775931078, "Y"=530129.3621610192}, {"X"=175272.4110996747, "Y"=530129.4009780311}, {"X"=175272.44518609784, "Y"=530129.4393815707}, {"X"=175272.4796800951, "Y"=530129.4772223142}, {"X"=175272.51379755183, "Y"=530129.5147367672}, {"X"=175272.5476820736, "Y"=530129.5513629087}, {"X"=175272.5806844585, "Y"=530129.5880282833}, {"X"=175272.61326672463, "Y"=530129.6243086737}, {"X"=175272.64593904302, "Y"=530129.6601881349}, {"X"=175272.6783208062, "Y"=530129.6966622323}, {"X"=175272.7108845465, "Y"=530129.7332678646}, {"X"=175272.74380051377, "Y"=530129.7697659085}, {"X"=175272.77675879907, "Y"=530129.8061961255}, {"X"=175272.80955542656, "Y"=530129.8424769914}, {"X"=175272.8417568801, "Y"=530129.8790836945}, {"X"=175272.87418592005, "Y"=530129.9153700864}, {"X"=175272.9071026067, "Y"=530129.9512133114}, {"X"=175272.9410808853, "Y"=530129.9871954591}, {"X"=175272.97502091975, "Y"=530130.0240234341}, {"X"=175273.00928738486, "Y"=530130.0616062572}, {"X"=175273.0438165611, "Y"=530130.0993636596}, {"X"=175273.07827987047, "Y"=530130.1370136032}, {"X"=175273.1123028364, "Y"=530130.1743285613}, {"X"=175273.14602526586, "Y"=530130.2109596252}, {"X"=175273.17947341292, "Y"=530130.2473972735}, {"X"=175273.21286651812, "Y"=530130.2837929111}, {"X"=175273.24664749746, "Y"=530130.3204537679}, {"X"=175273.2805465241, "Y"=530130.3580931731}, {"X"=175273.3147814621, "Y"=530130.3963986086}, {"X"=175273.35009392796, "Y"=530130.4348395892}, {"X"=175273.38586980384, "Y"=530130.4730283732}, {"X"=175273.42139343623, "Y"=530130.5109881624}, {"X"=175273.45635005386, "Y"=530130.5483125693}, {"X"=175273.49070351062, "Y"=530130.5853601836}, {"X"=175273.5242439296, "Y"=530130.6224479387}, {"X"=175273.55762271342, "Y"=530130.6590944481}, {"X"=175273.59098502202, "Y"=530130.6958608724}, {"X"=175273.6249620035, "Y"=530130.7329040531}, {"X"=175273.66006941308, "Y"=530130.7700004919}, {"X"=175273.69512346073, "Y"=530130.8073235014}, {"X"=175273.72971815502, "Y"=530130.8450718359}, {"X"=175273.76449848124, "Y"=530130.882391217}, {"X"=175273.79911156275, "Y"=530130.9194691412}, {"X"=175273.83402078584, "Y"=530130.9560445347}, {"X"=175273.86858358135, "Y"=530130.9925920963}, {"X"=175273.90292617198, "Y"=530131.029261284}, {"X"=175273.9374251662, "Y"=530131.0658001563}, {"X"=175273.97270876574, "Y"=530131.1022701154}, {"X"=175274.00795934038, "Y"=530131.139553701}, {"X"=175274.0435711147, "Y"=530131.1770681781}, {"X"=175274.0797913134, "Y"=530131.2139437965}, {"X"=175274.1158563591, "Y"=530131.2501739357}, {"X"=175274.150917573, "Y"=530131.2866267967}, {"X"=175274.18562281583, "Y"=530131.3228198938}, {"X"=175274.220102194, "Y"=530131.3593166493}, {"X"=175274.2555496864, "Y"=530131.3963932184}, {"X"=175274.29253605678, "Y"=530131.4344552332}, {"X"=175274.3302563675, "Y"=530131.474483967}, {"X"=175274.36883328803, "Y"=530131.515428021}, {"X"=175274.40837271762, "Y"=530131.5571516795}, {"X"=175274.4478430463, "Y"=530131.6003716328}, {"X"=175274.4872583938, "Y"=530131.6441699865}, {"X"=175274.52733322408, "Y"=530131.6878209964}, {"X"=175274.56796812185, "Y"=530131.7309564867}, {"X"=175274.6077128834, "Y"=530131.7738215836}, {"X"=175274.6455241114, "Y"=530131.816739013}, {"X"=175274.682436085, "Y"=530131.85809975}, {"X"=175274.71873880664, "Y"=530131.8971238163}, {"X"=175274.7533625209, "Y"=530131.9342050428}, {"X"=175274.7861236051, "Y"=530131.9695548476}, {"X"=175274.8175033924, "Y"=530132.0038898881}, {"X"=175274.84795043553, "Y"=530132.0370257078}, {"X"=175274.8780368938, "Y"=530132.0695388535}, {"X"=175274.90851497953, "Y"=530132.1026879033}, {"X"=175274.93991523306, "Y"=530132.1376532813}, {"X"=175274.97391482544, "Y"=530132.1745587783}, {"X"=175275.0098840713, "Y"=530132.2137414307}, {"X"=175275.04676271445, "Y"=530132.2546161485}, {"X"=175275.08410098526, "Y"=530132.2954573216}, {"X"=175275.12082564796, "Y"=530132.3351837915}, {"X"=175275.15588432993, "Y"=530132.3743780163}, {"X"=175275.1907411466, "Y"=530132.4127060378}, {"X"=175275.2257990393, "Y"=530132.450734913}, {"X"=175275.2611475317, "Y"=530132.4893833405}, {"X"=175275.29637687237, "Y"=530132.5293750499}, {"X"=175275.3316528765, "Y"=530132.5701701589}, {"X"=175275.36743519967, "Y"=530132.6108450161}, {"X"=175275.40344109156, "Y"=530132.650139658}, {"X"=175275.4383590333, "Y"=530132.6887704909}, {"X"=175275.47227939445, "Y"=530132.7270413497}, {"X"=175275.5063844877, "Y"=530132.7648777085}, {"X"=175275.54094360428, "Y"=530132.8037815187}, {"X"=175275.57606238793, "Y"=530132.8438301585}, {"X"=175275.61236367578, "Y"=530132.8844690769}, {"X"=175275.64928352344, "Y"=530132.9260994905}, {"X"=175275.68554765047, "Y"=530132.9679515942}, {"X"=175275.72036669948, "Y"=530133.0093851166}, {"X"=175275.75413836984, "Y"=530133.0494954524}, {"X"=175275.78700624986, "Y"=530133.0877139333}, {"X"=175275.8188459517, "Y"=530133.1248111655}, {"X"=175275.8501899214, "Y"=530133.1608155428}, {"X"=175275.88239211007, "Y"=530133.1964822053}, {"X"=175275.91512631148, "Y"=530133.2332282971}, {"X"=175275.948647906, "Y"=530133.2714459569}, {"X"=175275.98294943557, "Y"=530133.311010895}, {"X"=175276.01811435405, "Y"=530133.3510871474}, {"X"=175276.05312938656, "Y"=530133.390799809}, {"X"=175276.0877759427, "Y"=530133.4293193512}, {"X"=175276.12058547107, "Y"=530133.4672760782}, {"X"=175276.15208911267, "Y"=530133.5042577698}, {"X"=175276.1831761419, "Y"=530133.5399432683}, {"X"=175276.21427814369, "Y"=530133.5758995307}, {"X"=175276.24577882525, "Y"=530133.6127791256}, {"X"=175276.27912460643, "Y"=530133.6502548072}, {"X"=175276.313396601, "Y"=530133.6897177282}, {"X"=175276.3483805628, "Y"=530133.7309065964}, {"X"=175276.38374916016, "Y"=530133.7730621238}, {"X"=175276.4196610347, "Y"=530133.8156155951}, {"X"=175276.455288259, "Y"=530133.8586615745}, {"X"=175276.4907251926, "Y"=530133.9014606175}, {"X"=175276.52621986374, "Y"=530133.9440153224}, {"X"=175276.56167433667, "Y"=530133.985556844}, {"X"=175276.5958250264, "Y"=530134.026834746}, {"X"=175276.62880956824, "Y"=530134.0673624997}, {"X"=175276.66129835334, "Y"=530134.1061914169}, {"X"=175276.6935025365, "Y"=530134.1434329674}, {"X"=175276.72459505638, "Y"=530134.1794791566}, {"X"=175276.75498245785, "Y"=530134.2143176835}, {"X"=175276.78438415064, "Y"=530134.2492179489}, {"X"=175276.81322975375, "Y"=530134.2847802236}, {"X"=175276.84240576296, "Y"=530134.3209441777}, {"X"=175276.87308578577, "Y"=530134.3582845721}, {"X"=175276.90509450194, "Y"=530134.3974234485}, {"X"=175276.9385569887, "Y"=530134.4381229312}, {"X"=175276.97238543944, "Y"=530134.4803651446}, {"X"=175277.00645487237, "Y"=530134.5223225203}, {"X"=175277.0401530974, "Y"=530134.5630623702}, {"X"=175277.0730412123, "Y"=530134.6024350484}, {"X"=175277.10477501623, "Y"=530134.6405703183}, {"X"=175277.13569932047, "Y"=530134.6775448481}, {"X"=175277.16517660648, "Y"=530134.7134459837}, {"X"=175277.19316506683, "Y"=530134.7485135774}, {"X"=175277.22000726731, "Y"=530134.7826678182}, {"X"=175277.24660024542, "Y"=530134.8158172618}, {"X"=175277.27348351714, "Y"=530134.8485840561}, {"X"=175277.30092404727, "Y"=530134.880783176}, {"X"=175277.32825486694, "Y"=530134.9130259046}, {"X"=175277.3551759693, "Y"=530134.9454063558}, {"X"=175277.38202166307, "Y"=530134.9777459648}, {"X"=175277.4089487573, "Y"=530135.0097557076}, {"X"=175277.43556265638, "Y"=530135.041593237}, {"X"=175277.4623549861, "Y"=530135.0735612031}, {"X"=175277.4893954736, "Y"=530135.1061732625}, {"X"=175277.5171539628, "Y"=530135.1389596672}, {"X"=175277.54494050564, "Y"=530135.1722454247}, {"X"=175277.57209608817, "Y"=530135.2060369264}, {"X"=175277.59928448562, "Y"=530135.2392434345}, {"X"=175277.62629492726, "Y"=530135.27188111}, {"X"=175277.6531476071, "Y"=530135.3035891907}, {"X"=175277.679941679, "Y"=530135.3337503008}, {"X"=175277.70591114715, "Y"=530135.3636352749}, {"X"=175277.7306621187, "Y"=530135.3930410634}, {"X"=175277.7544783333, "Y"=530135.4220644931}, {"X"=175277.7785223435, "Y"=530135.4496399949}, {"X"=175277.80238363042, "Y"=530135.4768309147}, {"X"=175277.82533196377, "Y"=530135.5044229734}, {"X"=175277.84829750066, "Y"=530135.5324411679}, {"X"=175277.87154164902, "Y"=530135.5600201427}, {"X"=175277.8952151314, "Y"=530135.5878042838}, {"X"=175277.91869184974, "Y"=530135.6155501613}, {"X"=175277.94200009134, "Y"=530135.6429358316}, {"X"=175277.96469177437, "Y"=530135.6694076939}, {"X"=175277.98656638517, "Y"=530135.6945556883}, {"X"=175278.00726998152, "Y"=530135.717908063}, {"X"=175278.02607823673, "Y"=530135.7380507804}, {"X"=175278.04238282467, "Y"=530135.7544584541}, {"X"=175278.05608346884, "Y"=530135.7682667697}, {"X"=175278.0672667001, "Y"=530135.7781847019}, {"X"=175278.075528645, "Y"=530135.7839282118}, {"X"=175278.07986438635, "Y"=530135.7853526607}, {"X"=175278.08178297154, "Y"=530135.7829419246}, {"X"=175278.08224143783, "Y"=530135.778321333}, {"X"=175278.0817217421, "Y"=530135.7733174067}, {"X"=175278.08084463736, "Y"=530135.7687662473}, {"X"=175278.08048538852, "Y"=530135.7641014615}, {"X"=175278.08061412623, "Y"=530135.7585107199}, {"X"=175278.07962786822, "Y"=530135.7514937769}, {"X"=175278.07637335957, "Y"=530135.7421717034}, {"X"=175278.07053692619, "Y"=530135.7299083684}, {"X"=175278.06239563314, "Y"=530135.7137407054}, {"X"=175278.05169306954, "Y"=530135.6929303033}, {"X"=175278.03836551245, "Y"=530135.6674940016}, {"X"=175278.0221992266, "Y"=530135.639143834}, {"X"=175278.0041440234, "Y"=530135.6082587827}, {"X"=175277.98485462053, "Y"=530135.575177642}, {"X"=175277.96457856282, "Y"=530135.5400406278}, {"X"=175277.9434693148, "Y"=530135.5029216496}, {"X"=175277.92102088168, "Y"=530135.4634515083}, {"X"=175277.8966213828, "Y"=530135.4216986073}, {"X"=175277.87026081482, "Y"=530135.3766763115}, {"X"=175277.8418635917, "Y"=530135.3279864021}, {"X"=175277.81099544337, "Y"=530135.2770474545}, {"X"=175277.7777387605, "Y"=530135.2238636677}, {"X"=175277.7424477724, "Y"=530135.1687059047}, {"X"=175277.70587482766, "Y"=530135.1113788285}, {"X"=175277.6688537235, "Y"=530135.0513727687}, {"X"=175277.63116314998, "Y"=530134.9890346522}, {"X"=175277.59250670258, 
